vi "[GV]_GPS Raw_Speed.vi"() -> ()   [LabVIEW 2016]
panel:
  out "GPS Raw_Speed (m/s)":dbl format="%.2g"
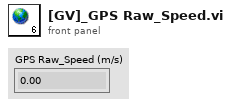
[diagram p1: front panel]
diagram:
